vi "MultiColumnListbox_ColorRows.vi"(7 "Parent VI Reference":refnum<vi>, 8 "error in":errorcluster, 9 "Color Odd Rows":u32(colorbox)=16120574, 10 "Color Even Rows":u32(colorbox)=16448250, 11 "MCListbox Refnum":refnum<vi>) -> (0 "error out":errorcluster)   [LabVIEW 2022 SP3, in "hse-ui.lvlib"]
doc: "Colors the rows of a MCLB in alternate colors. If <b>Parent VI Reference</b> is supplied, panel updates are deferred.\n\n____\nHAMPEL SOFTWARE ENGINEERING v3.8.0 (2023-12-18 14:41)"
uses:
  hse-ui.lvlib
  <vilib>/Utility/miscctls.llb/LVRowAndColumnTypeDef.ctl
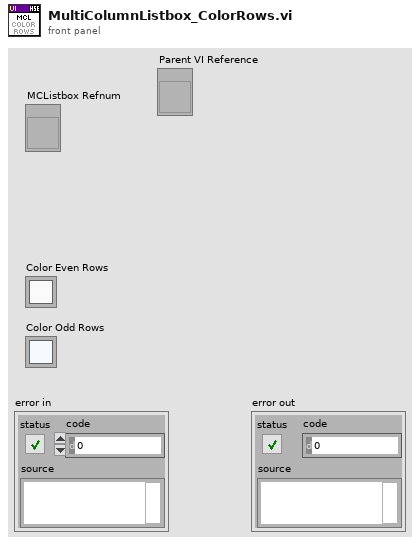
[diagram p1: front panel]
types:
  T1 = typedef "LVRowAndColumnTypeDef.ctl" = cluster{"Row":i32, "Column":i32}
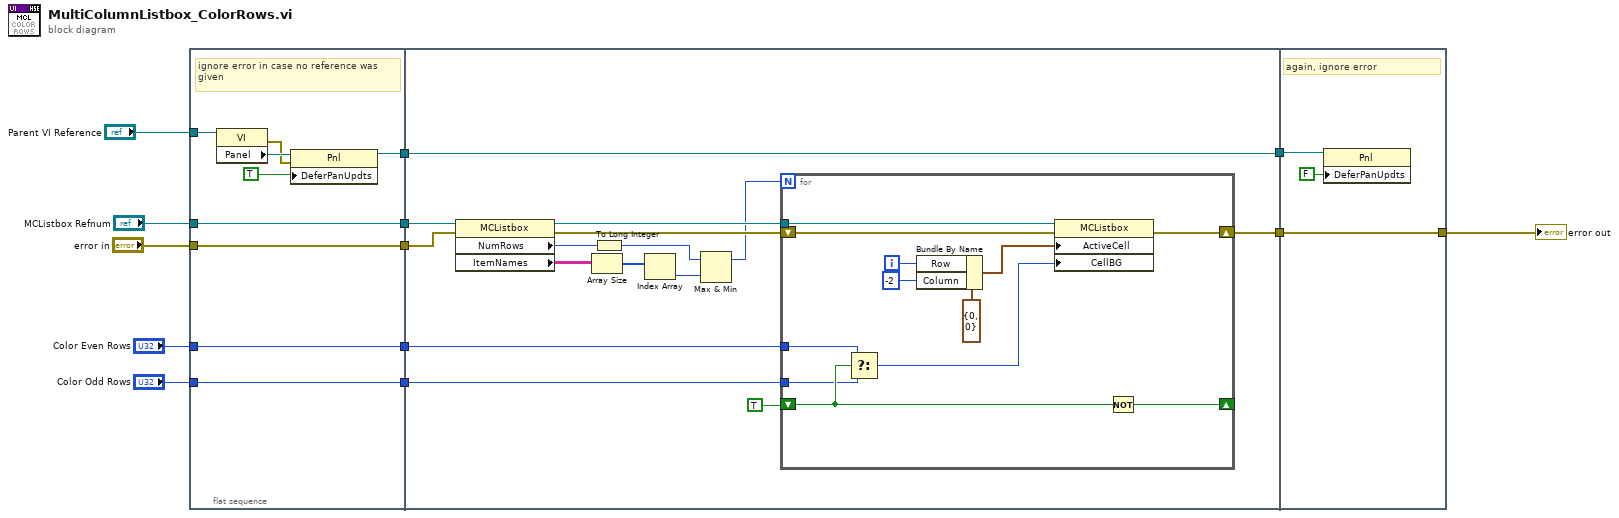
[diagram p0: block diagram]
diagram:
  n1 = flat-sequence {
    tunnel: "MCListbox Refnum" -> [w22]
    tunnel: [w22] -> w13
    tunnel: [w18] -> w12
    tunnel: "error in" -> [w18]
    tunnel: "Parent VI Reference" -> [w17]
    tunnel: [w16] -> w9
    tunnel: "Color Even Rows" -> [w15]
    tunnel: [w15] -> w4
    tunnel: "Color Odd Rows" -> [w14]
    tunnel: [w14] -> w2
    tunnel: w13 -> [w29]
    tunnel: w12 -> [w27]
    tunnel: w9 -> [w26]
    tunnel: [w28] -> w8
    tunnel: [w26] -> w7
    tunnel: w4 -> [w25]
    tunnel: w2 -> [w24]
    tunnel: [w52] -> w6
    tunnel: w8 -> [w52]
    tunnel: w7 -> [w50]
    frame #0 {
      # "ignore error in case no reference was given"
      n2 = property class="VI"(reference=w17) -> (error out=w20:errorcluster, "Panel"=w21:refnum<vi>)  [unwired: 1 in, 1 out]
      n3 = property class="Pnl"(reference=w21, error in=w20, "DeferPanUpdts"=TRUE ("Defer Panel Updates")) -> (reference out=w16:refnum<vi>)  [unwired: 1 out]
    }
    frame #1 {
      n4 = property on="Property Node" class="MCListbox"(reference=w29, error in=w27) -> (reference out=w32:refnum<vi>, error out=w31:errorcluster, "NumRows"=w33:u32, "ItemNames"=w34:string[][])
      n5 = Array Size(array=w34) -> (size(s)=w37:i32[])
      n6 = To Long Integer(number=w33) -> (32bit integer=w23:i32)
      n7 = Index Array(array=w37) -> (element=w36:i32)  [unwired: 1 in]
      n8 = Max & Min(x=w23, y=w36) -> (max(x,y)=w30:i32)  [unwired: 1 out]
      n9 = for {
        N: w30 -> [_]
        shift-right: [w45] -> _
        shift-left: TRUE -> [w44]
        tunnel: w32 -> [w42]
        shift-right: [w40] -> w28
        shift-left: w31 -> [w41]
        tunnel: w25 -> [w39]
        tunnel: w24 -> [w38]
        i -> [w47]
        n10 = Select(t=w39, s=w44, f=w38) -> (s? t:f=w43:u32)
        n11 = Bundle By Name(cluster=T1 {"Row"=0, "Column"=0} ("Active Cell:Active Cell"), "Row"=w47, "Column"=-2) -> (w48:T1)
        n12 = property on="Property Node" class="MCListbox"(reference=w42, error in=w41, "ActiveCell"=w48, "CellBG"=w43) -> (error out=w40:errorcluster)  [unwired: 1 out]
        n13 = Not(x=w44) -> (.not. x?=w45:bool)
      }
    }
    frame #2 {
      # "again, ignore error"
      n14 = property class="Pnl"(reference=w50, "DeferPanUpdts"=FALSE ("Defer Panel Updates")) -> ()  [unwired: 1 in, 2 out]
    }
  }
  "error out" <- w6
